vi "Auto Match.vi"() -> ()   [LabVIEW 2012]
doc: "本VI演示了通过隧道将数据传递出While循环。该VI将连续生成随机数，直到生成数字与指定数字相匹配为止。计数接线端记录了匹配发生前的循环次数。"
panel:
  out "循环计数":i32
  out "当前数":u32 format="%#.0f"
  in  "待匹配数字":u32=50 max=1000 step=1
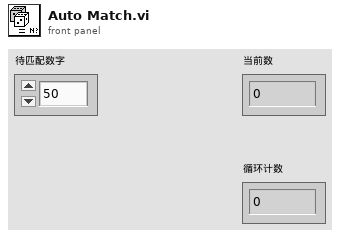
[diagram p1: front panel]
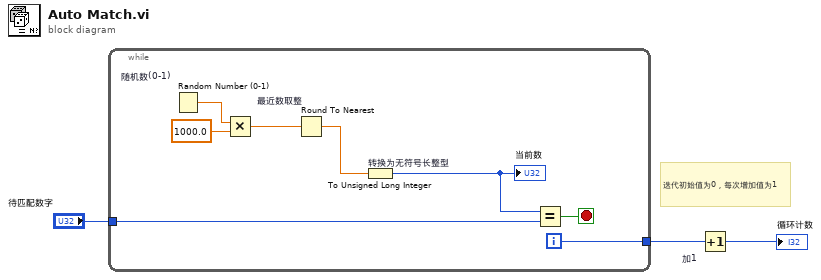
[diagram p0: block diagram]
diagram:
  # "迭代初始值为0，每次增加值为1"
  n1 = while {
    tunnel: [w7] -> w3
    tunnel: "待匹配数字" -> [w6]
    i -> [w7]
    stop <- w8 stop-if-true
    n2 = Random Number (0-1) "随机数(0-1)"() -> (number: 0 to 1=w9:dbl)
    n3 = Multiply ("乘")(x=w9, y=1000.0) -> (x*y=w11:dbl)
    n4 = Round To Nearest "最近数取整"(number=w11) -> (nearest integer value=w5:dbl)
    n5 = To Unsigned Long Integer "转换为无符号长整型"(number=w5) -> (unsigned 32bit integer=w4:u32)
    "当前数" <- w4
    n6 = Equal? ("等于？")(x=w4, y=w6) -> (x = y?=w8:bool)
  }
  n7 = Increment "加1"(x=w3) -> (x+1=→"循环计数":i32)
